vi "HideShowFrontPanel.vi"(7 "Operation":T1=enum."Hide 80%", 8 "Error In":errorcluster, 11 "VI Name Or Path (Caller)":string) -> (0 "Error Out":errorcluster)   [LabVIEW 2011]
uses:
  Controls/TransparencyEffectOperations.ctl
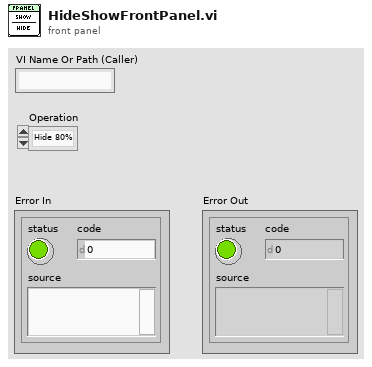
[diagram p1: front panel]
types:
  T1 = typedef "TransparencyEffectOperations.ctl" = enum16{"Show", "Hide 80%", "Hide All"}
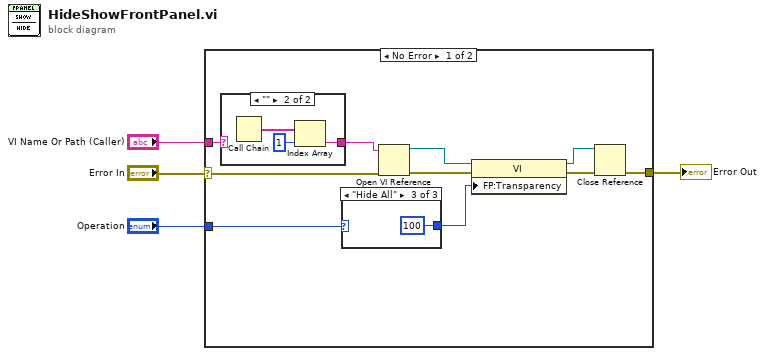
[diagram p0: block diagram]
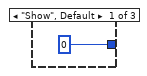
[diagram p3: hidden frame]
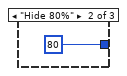
[diagram p4: hidden frame]
diagram:
  n1 = case shown="No Error" "Error In" {
    selector: "Error In" -> [w7 w22]
    tunnel: "Operation" -> [w12 _]
    tunnel: [w8 w22] -> w3
    tunnel: "VI Name Or Path (Caller)" -> [w5 _]
    frame No Error {
      n2 = case shown="\"\"" w5 {
        selector: w5 -> [w15 _]
        tunnel: [w15 w17] -> w6
        frame Default {
        }
        frame "" {
          n3 = Call Chain() -> (call chain=w18:string[])
          n4 = Index Array(array=w18, index=1) -> (element=w17:string)
        }
      }
      n5 = case shown="\"Hide All\"" w12 {
        tunnel: [0 80 100] -> w11
        frame "Show", Default {
        }
        frame "Hide 80%" {
        }
        frame "Hide All" {
        }
      }
      n6 = Open VI Reference(vi path=w6, error in (no error)=w7) -> (vi reference=w14:refnum<vi>, error out=w13:errorcluster)  [unwired: 4 in]
      n7 = property class="VI"(reference=w14, error in=w13, "FP:Transparency"=w11) -> (reference out=w9:refnum<vi>, error out=w10:errorcluster)
      n8 = Close Reference(reference=w9, error in (no error)=w10) -> (error out=w8:errorcluster)
    }
    frame Error {
    }
  }
  "Error Out" <- w3
